vi "Build Register Status Message.vi"(0 "CSM Name":string, 5 "Source CSM Name (* as Default)":string="*", 7 "Status":string, 9 "Response Message (if \"\", same as Source Message)":string) -> (6 "State with Arguments":string)   [LabVIEW 2020, in "Communicable State Machine.lvlib"]
doc: "Builds register status message. The message looks like:\n[source-state]@[source-module] >> [response-message]@[response-module] -><register>\nFor examples:\nDownloadFinished@Downloader >> StartPlay@Player -><register>\nDownloadFinished@Downloader >> StartPlay -><register> // response-module is current module\nDownloadFinished@Downloader -><register> // response-module is current module. response-message is DownloadFinished\nDownloadFinished@* >> StartPlay@Player -><register> // Any Module's DownloadFinished is registered to Player's StartPlay state.\n\n<b>Inputs:</b>\n - <b>Source CSM Name (* as Default)</b>:\n - <b>CSM Name</b>:\n - <b>Status</b>:\n - <b>Response Message (if \"\", same as Source Message)</b>:\n\n<b>Outputs:</b>\n - <b>State with Arguments</b>:"
uses:
  Communicable State Machine.lvlib
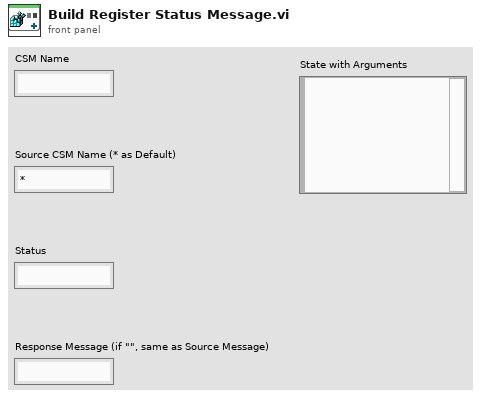
[diagram p1: front panel]
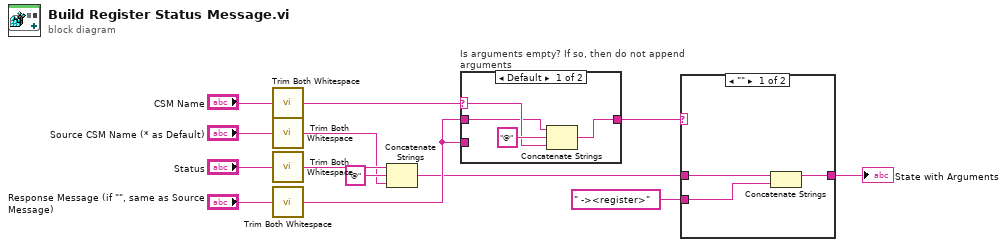
[diagram p0: block diagram]
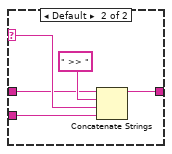
[diagram p2: hidden frame]
diagram:
  n1 = call "Trim Both Whitespace.vi"("string"="CSM Name") -> ("trimmed string"=w4:string)  [unwired: 1 in]
  n2 = call "Trim Both Whitespace.vi"("string"="Source CSM Name (* as Default)") -> ("trimmed string"=w6:string)  [unwired: 1 in]
  n3 = call "Trim Both Whitespace.vi"("string"="Status") -> ("trimmed string"=w8:string)  [unwired: 1 in]
  n4 = call "Trim Both Whitespace.vi"("string"="Response Message (if \"\", same as Source Message)") -> ("trimmed string"=w5:string)  [unwired: 1 in]
  n5 = Concatenate Strings(w8, "@" ("string"), w6) -> (w2:string)
  n6 = case "Is arguments empty? If so, then do not append arguments" shown="Default" w4 {
    selector: w4 -> [w15 _]
    tunnel: [w16 w18] -> w3
    tunnel: w5 -> [w14 w18]
    tunnel: w5 -> [_ _]
    frame Default {
      n7 = Concatenate Strings(w14, "@" ("string"), w15) -> (w16:string)
    }
    frame "" {
    }
  }
  n8 = case shown="\"\"" w3 {
    selector: w3 -> [_ w24]
    tunnel: [w19 w26] -> w13
    tunnel: w2 -> [w21 w23]
    tunnel: " -><register>" ("string") -> [w20 w22]
    frame "" {
      n9 = Concatenate Strings(w21, w20) -> (w19:string)
    }
    frame Default {
      n10 = Concatenate Strings(w23, " >> " ("string"), w24, w22) -> (w26:string)
    }
  }
  "State with Arguments" <- w13
